vi "Exp_SetExperiment.vi"(8 "error in (no error)":errorcluster, 10 "ExperimentName":string, 11 "LightField Automation in":refnum<class "LightField Automation.lvclass">) -> (0 "error out":errorcluster, 3 "LightField Automation out":refnum<class "LightField Automation.lvclass">)   [LabVIEW 2013, in "LightField Automation.lvclass"]
uses:
  LightField Automation.lvclass
  LightField Automation.lvclass/LightField Automation.ctl
  C:/Program Files/Princeton Instruments/LightField/AddInViews/PrincetonInstruments.LightFieldViewV3.dll
  Program Files/Princeton Instruments/LightField/AddInViews/PrincetonInstruments.LightFieldViewV3.dll
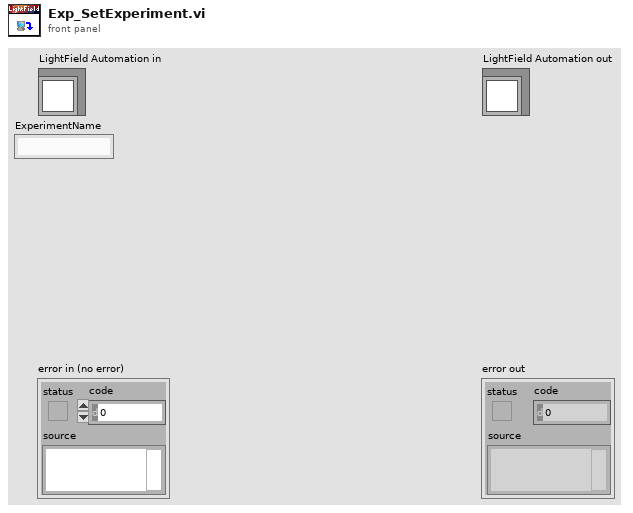
[diagram p1: front panel]
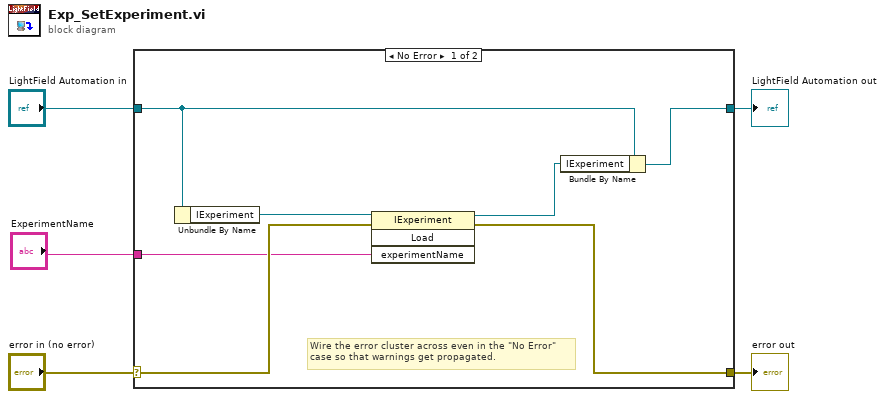
[diagram p0: block diagram]
diagram:
  n1 = case shown="No Error" "error in (no error)" {
    selector: "error in (no error)" -> [w11 w14]
    tunnel: [w10 w14] -> w4
    tunnel: [w7 w13] -> w2
    tunnel: "LightField Automation in" -> [w8 w13]
    tunnel: "ExperimentName" -> [w9 _]
    frame No Error {
      # "Wire the error cluster across even in the \"No Error\"\ncase so that warnings get propagated."
      n2 = Unbundle By Name(w8) -> ("IExperiment"=w12:refnum<k24>)
      n3 = invoke class="IExperiment" method="Load"(reference=w12, error in=w11, "experimentName"=w9) -> (reference out=w6:refnum<k24>, error out=w10:errorcluster)  [unwired: 1 in, 2 out]
      n4 = Bundle By Name(cluster=w8, "IExperiment"=w6) -> (w7:refnum<class "LightField Automation.lvclass">)
    }
    frame Error {
    }
  }
  "error out" <- w4
  "LightField Automation out" <- w2
